vi "ReadDataFifo.vi"(8 "error in (no error)":errorcluster, 11 "PmuBase in":refnum<class "PmuBase.lvclass">) -> (0 "error out":errorcluster, 3 "PmuBase out":refnum<class "PmuBase.lvclass">)   [LabVIEW 2018, in "SensorPlugins.lvlib" / "PmuBase.lvclass"]
uses:
  PmuBase.lvclass
  Typedef/PmuData.ctl
  PmuBase.lvclass/PmuBase.ctl
  Accessors/Write DataFifo.vi
  Accessors/Read PmuDataArray.vi
  Accessors/Read DataFifo.vi
panel:
  out "PmuReport":T1 {"Synx" format="%#_4g"}
  out "DataValid":bool
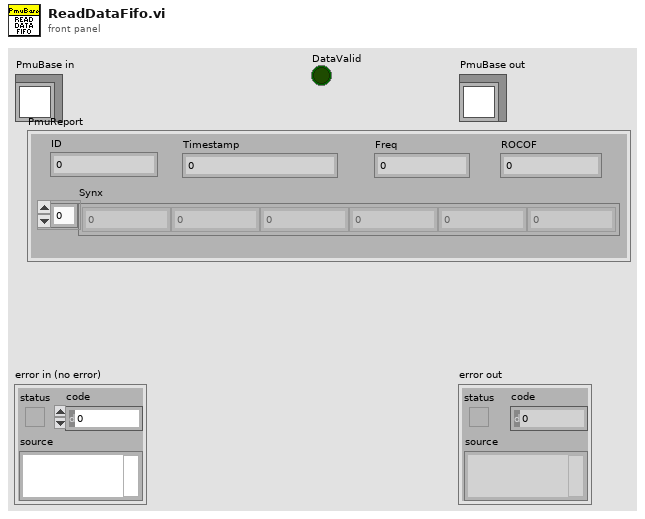
[diagram p1: front panel]
types:
  T1 = typedef "SensorPlugins.lvlib/PmuBase.lvclass/PmuData.ctl" = cluster{"Timestamp":dbl, "Synx":cdb[], "Freq":dbl, "ROCOF":dbl, "ID":i16}
  T2 = typedef "DataFifo.ctl" = cluster{"ReadPointer":u16, "WritePointer":u64, "Locked":bool, "FifoSize":u64}
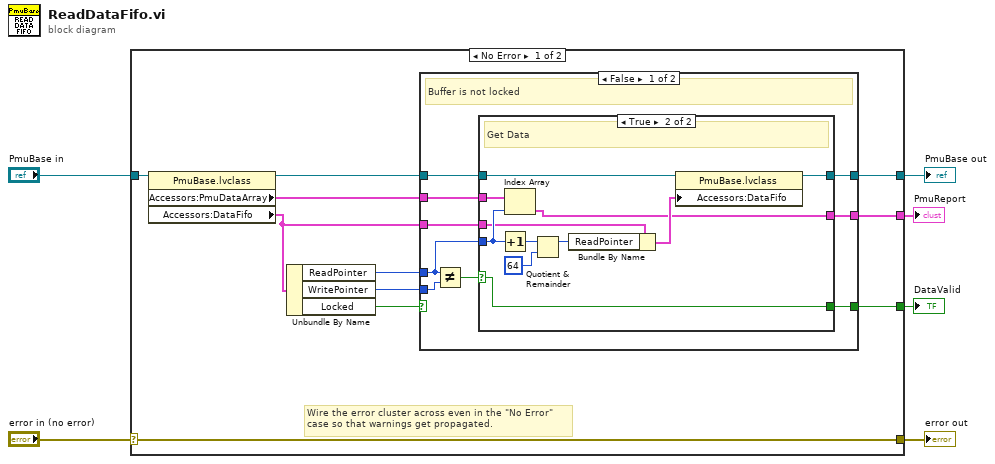
[diagram p0: block diagram]
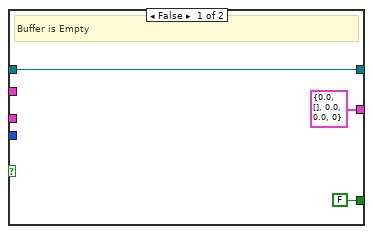
[diagram p2: hidden frame]
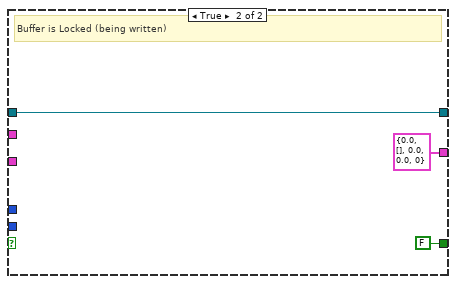
[diagram p3: hidden frame]
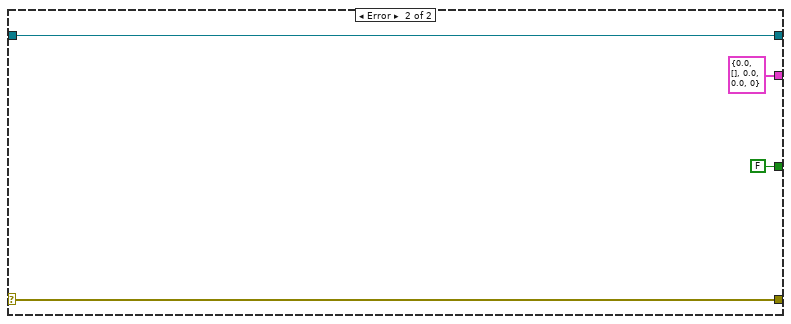
[diagram p4: hidden frame]
diagram:
  n1 = case shown="No Error" "error in (no error)" {
    selector: "error in (no error)" -> [w16 w47]
    tunnel: [w16 w47] -> w5
    tunnel: [w9 w46] -> w3
    tunnel: "PmuBase in" -> [w17 w46]
    tunnel: [w14 FALSE] -> w2
    tunnel: [w7 T1 {"Timestamp"=0.0, "Synx"=[], "Freq"=0.0, "ROCOF"=0.0, "ID"=0} ("PmuReport")] -> w1
    frame No Error {
      # "Wire the error cluster across even in the \"No Error\"\ncase so that warnings get propagated."
      n2 = property class="PmuBase.lvclass"(reference=w17) -> (reference out=w10:refnum<class "PmuBase.lvclass">, "Accessors:PmuDataArray"=w11:T1[], "Accessors:DataFifo"=w8:T2)  [unwired: 1 in, 1 out]
      n3 = Unbundle By Name(w8) -> ("ReadPointer"=w12:u16, "WritePointer"=w13:u64, "Locked"=w15:bool)
      n4 = case shown="False" w15 {
        tunnel: [w25 FALSE] -> w14
        tunnel: w13 -> [w24 _]
        tunnel: w12 -> [w20 _]
        tunnel: w11 -> [w23 _]
        tunnel: w10 -> [w22 w43]
        tunnel: [w21 w43] -> w9
        tunnel: w8 -> [w19 _]
        tunnel: [w18 T1 {"Timestamp"=0.0, "Synx"=[], "Freq"=0.0, "ROCOF"=0.0, "ID"=0} ("PmuReport")] -> w7
        frame False {
          # "Buffer is not locked"
          n5 = Not Equal?(x=w20, y=w24) -> (x != y?=w26:bool)
          n6 = case shown="True" w26 {
            selector: w26 -> [_ w40]
            tunnel: [FALSE w40] -> w25
            tunnel: w23 -> [_ w38]
            tunnel: w22 -> [w29 w39]
            tunnel: [w29 w34] -> w21
            tunnel: w20 -> [_ w37]
            tunnel: w19 -> [_ w33]
            tunnel: [T1 {"Timestamp"=0.0, "Synx"=[], "Freq"=0.0, "ROCOF"=0.0, "ID"=0} ("PmuReport") w30] -> w18
            frame False {
              # "Buffer is Empty"
            }
            frame True {
              # "Get Data"
              n7 = Increment(x=w37) -> (x+1=w36:u16)
              n8 = Index Array(array=w38, index=w37) -> (element=w30:T1)
              n9 = Quotient & Remainder(x=w36, y=i8 64) -> (x-y*floor(x/y)=w32:u16)  [unwired: 1 out]
              n10 = Bundle By Name(cluster=w33, "ReadPointer"=w32) -> (w31:T2)
              n11 = property class="PmuBase.lvclass"(reference=w39, "Accessors:DataFifo"=w31) -> (reference out=w34:refnum<class "PmuBase.lvclass">)  [unwired: 1 in, 1 out]
            }
          }
        }
        frame True {
          # "Buffer is Locked (being written)"
        }
      }
    }
    frame Error {
    }
  }
  "error out" <- w5
  "PmuBase out" <- w3
  "DataValid" <- w2
  "PmuReport" <- w1
